vi "Read Display Format.vi"(8 "error in":errorcluster, 9 "form in":T1, 10 "precision in":i32, 11 "PV Data in":refnum<class "PV Data.lvclass">) -> (0 "error out":errorcluster, 1 "form":T1, 2 "precision":i32, 3 "PV Data out":refnum<class "PV Data.lvclass">)   [LabVIEW 2020, in "PV Access.lvlib" / "PV Data.lvlib" / "PV Data.lvclass"]
uses:
  PV Data.lvclass
  PV Access.lvlib
  Display Form.ctl
  PV Data.lvlib
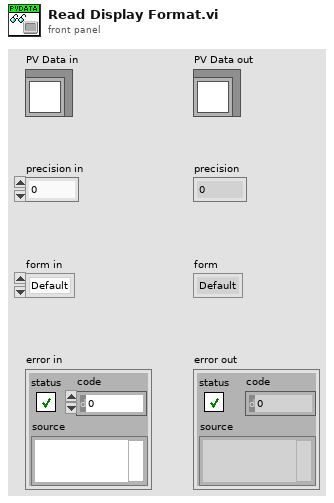
[diagram p1: front panel]
types:
  T1 = typedef "PV Access.lvlib/PV Data.lvlib/Display Form.ctl" = enum32{"Default", "String", "Binary", "Decimal", "Hex", "Exponential", "Engineering"}
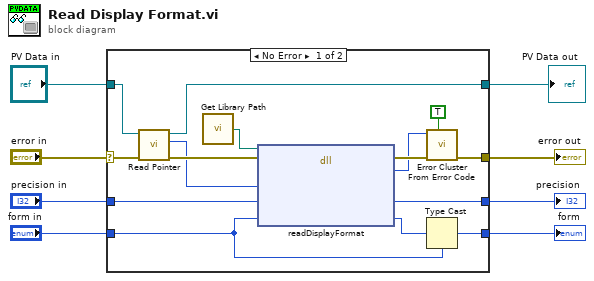
[diagram p0: block diagram]
diagram:
  n1 = case shown="No Error" "error in" {
    selector: "error in" -> [w18 w27]
    tunnel: [w19 w27] -> w8
    tunnel: "PV Data in" -> [w16 w26]
    tunnel: [w14 w26] -> w5
    tunnel: [w13 w24] -> w4
    tunnel: [w10 w25] -> w3
    tunnel: "precision in" -> [w12 w24]
    tunnel: "form in" -> [w9 w25]
    frame No Error {
      n2 = call-dynamic "Read Pointer.vi"("error in (no error)"=w18, "Pointer Base in"=w16) -> ("error out"=w17:errorcluster, "Pointer"=w15:i64, "Pointer Base out"=w14:refnum<class "PV Data.lvclass">)  [unwired: 7 in]
      n3 = call "Get Library Path.vi"() -> ("Path"=w23:path)  [unwired: 1 in]
      n4 = dll-call lib="?" fn="readDisplayFormat"(path in=w23, error in=w17, "value"=w15, "precision"=w12, "display metadata"=w9) -> (error out=w21:errorcluster, "err_code"=w20:i32, "precision"=w13:i32, "display metadata"=w11:i32)  [unwired: 2 in, 1 out]
      n5 = call <vilib>:"Error Cluster From Error Code.vi"("show call chain? (False)"=TRUE, "error in (no error)"=w21, "error code (0)"=w20) -> ("error out"=w19:errorcluster)  [unwired: 6 in]
      n6 = Type Cast(type=w9, x=w11) -> (*(type *) &x=w10:T1)
    }
    frame Error {
    }
  }
  "error out" <- w8
  "PV Data out" <- w5
  "precision" <- w4
  "form" <- w3
